vi "Create Request.vi"(6 "timeout (0 = Use Default)":i32, 8 "error in (no error)":errorcluster, 9 "Path":string, 10 "request specific headers":T1[](array[typedef]), 11 "REST Client in":refnum<class "REST Client.lvclass">) -> (0 "error out":errorcluster, 1 "Resolved URL":string, 2 "http-client":refnum<class "http-client.lvclass">, 3 "REST Client out":refnum<class "REST Client.lvclass">, 5 "Timeout":i32)   [LabVIEW 2020, in "REST Client.lvlib" / "REST Client.lvclass"]
uses:
  REST Client.lvclass
  REST Client.lvclass/REST Client.ctl
  http-client/http-client.lvclass
  HTTP Header.ctl
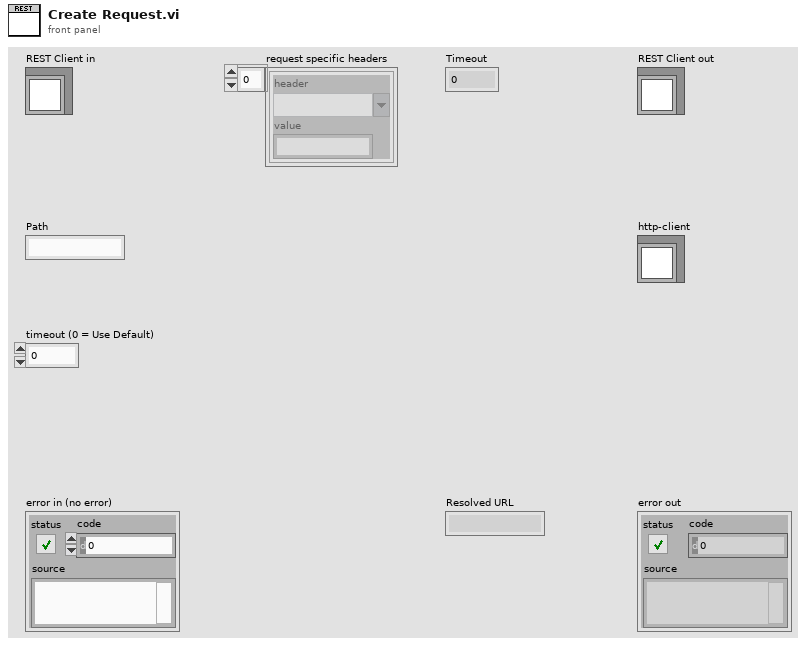
[diagram p1: front panel]
types:
  T1 = typedef "REST Client.lvlib/REST Client.lvclass/HTTP Header.ctl" = cluster{"header":string, "value":string}
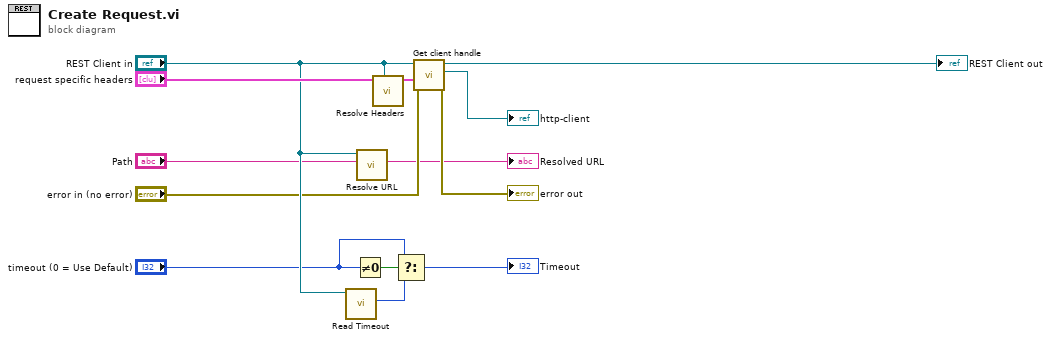
[diagram p0: block diagram]
diagram:
  n1 = call-dynamic "Read Timeout.vi"("REST Client in"="REST Client in") -> ("Timeout"=w8:i32)  [unwired: 8 in, 2 out]
  n2 = Not Equal To 0?(x="timeout (0 = Use Default)") -> (x != 0?=w4:bool)
  n3 = call "Resolve URL.vi"("Path"="Path", "REST Client in"="REST Client in") -> ("Resolved URL"=→"Resolved URL":string)  [unwired: 9 in]
  n4 = call "Resolve Headers.vi"("REST Client in"="REST Client in", "headers in"="request specific headers") -> ("headers out"=w12:T1[])  [unwired: 9 in]
  n5 = Select(t="timeout (0 = Use Default)", s=w4, f=w8) -> (s? t:f=→"Timeout":i32)
  n6 = call "Get client handle.vi"("error in (no error)"="error in (no error)", "headers"=w12, "REST Client in"="REST Client in") -> ("error out"=→"error out":errorcluster, "http-client"=→"http-client":refnum<class "http-client.lvclass">, "REST Client out"=→"REST Client out":refnum<class "REST Client.lvclass">)  [unwired: 6 in]
